vi "terminate.vi"(8 "error in (no error)":errorcluster, 11 "GenericPlugin in":refnum<class "ScanHeadMH100729FPGA.lvclass">) -> (0 "error out":errorcluster, 3 "GenericPlugin out":refnum<class "ScanHeadMH100729FPGA.lvclass">)   [LabVIEW 2010, in "ScanHeadMH100729FPGA.lvclass"]
doc: "The dynamic dispatch version of this VI terminates the plug-in object by releasing all of its resources."
uses:
  ScanHeadMH100729FPGA.lvclass
  AnalogOut/GenericAnalogOut/GenericAnalogOut/GenericAnalogOut.lvclass
  GenericScanHead/GenericScanHead/GenericScanHead.lvclass
  common/classes/ErrorController/ErrorController/class_data.vi
  common/classes/ErrorController/ErrorController/ErrorController.lvclass
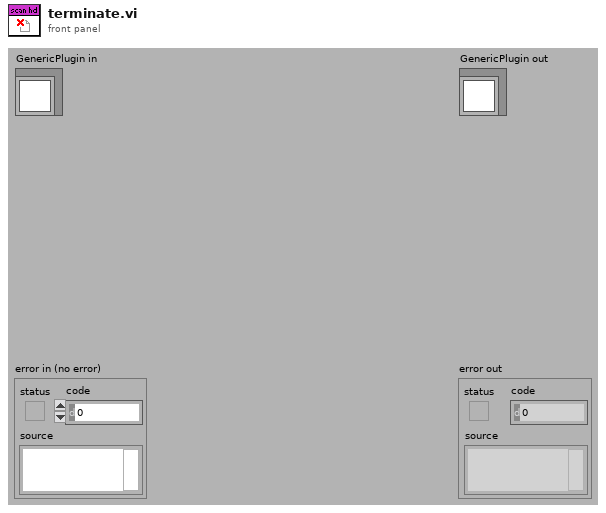
[diagram p1: front panel]
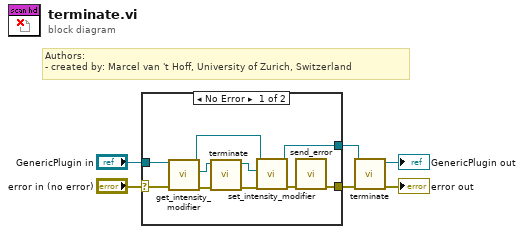
[diagram p0: block diagram]
diagram:
  # "Authors: \n- created by: Marcel van 't Hoff, University of Zurich, Switzerland"
  n1 = case shown="No Error" "error in (no error)" {
    selector: "error in (no error)" -> [w15 w18]
    tunnel: [w16 w18] -> w3
    tunnel: [w7 w17] -> w2
    tunnel: "GenericPlugin in" -> [w14 w17]
    frame No Error {
      n2 = call-dynamic "get_intensity_modifier.vi"("error in (no error)"=w15, "ScanHeadMH100729FPGA in"=w14) -> ("error out"=w13:errorcluster, "intensity modifier"=w12:refnum<class "GenericAnalogOut.lvclass">, "ScanHeadMH100729FPGA out"=w8:refnum<class "ScanHeadMH100729FPGA.lvclass">)  [unwired: 7 in]
      n3 = call-dynamic "terminate.vi"("error in (no error)"=w13, "GenericPlugin in"=w12) -> ("error out"=w11:errorcluster, "GenericPlugin out"=w9:refnum<class "GenericAnalogOut.lvclass">)  [unwired: 8 in]
      n4 = call-dynamic "set_intensity_modifier.vi"("error in (no error)"=w11, "intensity modifier"=w9, "ScanHeadMH100729FPGA in"=w8) -> ("error out"=w10:errorcluster, "ScanHeadMH100729FPGA out"=w7:refnum<class "ScanHeadMH100729FPGA.lvclass">)  [unwired: 7 in]
      n5 = call "send_error.vi"("error in (no error)"=w10) -> ("error out"=w16:errorcluster)  [unwired: 10 in]
    }
    frame Error {
    }
  }
  n6 = call-parent "terminate.vi"("error in (no error)"=w3, "GenericPlugin in"=w2) -> ("error out"=→"error out":errorcluster, "GenericPlugin out"=→"GenericPlugin out":refnum<class "ScanHeadMH100729FPGA.lvclass">)  [unwired: 8 in]
